vi "Fpga-FPGANic-Top.vi"() -> ()   [LabVIEW 2018]
uses:
  <instrlib>/_niInstr/Network/Ethernet/MAC/CLIP/v1/Resources.ctl
  <vilib>/Platform/TimedLoop/XDataNode/timing_clust.ctl
  <vilib>/Platform/TimedLoop/XDataNode/nitl_modes.ctl
  <vilib>/Platform/TimedLoop/XDataNode/wakeup.ctl
  <instrlib>/_niInstr/Network/Ethernet/MAC/Raw Stream/v1/niInstr Ethernet MAC Raw Stream v1.lvclass
  <instrlib>/_niInstr/Network/Ethernet/Utility/v1/FPGA/Network Data Stream.ctl
  States/FPGANic.Read.States.ctl
  States/FPGANic.Write.States.ctl
  <vilib>/rvi/Emulation/niFpgaSctlEmulationGetInTimedLoop.vi
  <vilib>/rvi/Emulation/niFpgaEmulationReportErrorSimple.vi
  <vilib>/rvi/Emulation/niFpgaGetClockAttributes.vi
  <vilib>/rvi/Emulation/niFpgaCriticalErrorInLSC.vi
  <vilib>/rvi/eio/common/nirviEmuTemplateMethod_errors.vi
  <vilib>/rvi/interface/RandomDataEmulation/niFpgaRandomDataHandleErrors.vi
  <vilib>/rvi/DataTransferAndStorage/Container/Common/niFpgaContainerGetUniqueNameForEmu.vi
  <vilib>/rvi/DataTransferAndStorage/Container/Common/niFpgaContainerSetEmuInfo.vi
  <vilib>/rvi/eio/common/nirviEmuReportErrorAndStop.vi
  <vilib>/rvi/DataTransferAndStorage/Container/Common/niFpgaContainerExecOnDevCompGetState.vi
  <vilib>/rvi/Emulation/niFpgaEmulationIsFPGAContextNoSignature.vi
  <vilib>/rvi/errors/niFpgaSetErrorForExecOnDevCompSimple.vi
  <vilib>/rvi/FIFO/Fifo_Resource/nirvififoEmulationSetSize.vi
  <vilib>/rvi/FIFO/Fifo_Resource/nirviFifoEmulationQueueMgr.vi
  <instcachedir>/0/nirviFifoEmulationQueueMgr_E5CAEC123FF24DC58D834DCA3CDAA9B5.lvgen/nirviFifoEmulationQueueMgr_E5CAEC123FF24DC58D834DCA3CDAA9B5_003.vi
  <vilib>/rvi/FIFO/Fifo_Resource/nirvififoEmulationDetermineInputValidOut.vi
  <vilib>/rvi/FIFO/Fifo_Resource/nirvififoEmulationCreateLock.vi
  <vilib>/rvi/Emulation/niFpgaProcessEmulError.vi
  <vilib>/rvi/FIFO/Fifo_Resource/nirvififoEmulationObtainLock.vi
  <vilib>/rvi/FIFO/Fifo_Resource/nirvififoEmulationReleaseLock.vi
  <vilib>/rvi/occurrence/nirviWaitOnOccurrenceBase.vi
  <vilib>/rvi/errors/nirviReportUnexpectedCaseInternalError.vi
  <vilib>/rvi/errors/nirviReportUnexpectedCaseInternalError (U32).vi
  <vilib>/Utility/error.llb/Clear Errors.vi
  <instrlib>/_niInstr/Network/Ethernet/MAC/Raw Stream/v1/Read End of Bad Frame.vi
  <instrlib>/_niInstr/Network/Ethernet/MAC/Raw Stream/v1/Read End of Good Frame.vi
  <instrlib>/_niInstr/Network/Ethernet/MAC/Raw Stream/v1/Read Data Stream.vi
  <instcachedir>/0/nirviFifoEmulationQueueMgr_E5CAEC123FF24DC58D834DCA3CDAA9B5.lvgen/nirviFifoEmulationQueueMgr_E5CAEC123FF24DC58D834DCA3CDAA9B5_006.vi
  <instrlib>/_niInstr/Network/Ethernet/MAC/Raw Stream/v1/Write Data Stream.vi
  <instrlib>/_niInstr/Network/Ethernet/MAC/Raw Stream/v1/Write End of Bad Frame.vi
  <instrlib>/_niInstr/Network/Ethernet/MAC/Raw Stream/v1/Write End of Good Frame.vi
  <vilib>/Platform/TimedLoop/XDataNode/XDataNode.xnode
  <vilib>/eio/EIONode/EIONode.xnode
  <vilib>/rvi/DataTransferAndStorage/Container/XNode/niFpgaContainer.xnode
  <vilib>/rvi/interface/RandomDataEmulation/nirviRandomDataFpgaReadWriteTemplate.vi
  <vilib>/rvi/LocalResourceManager/LocalResourceManager.xnode
  <vilib>/rvi/FIFO/Fifo_Resource/niFpgaFifoEmulationRefIn.vi
  <instrlib>/_niInstr/Network/Ethernet/MAC/CLIP/v1/niInstr Ethernet MAC - CLIP v1.lvclass
  <vilib>/Platform/TimedLoop/XDataNode/XDNodeRunTimeDep.lvlib
  <instrlib>/_niInstr/Network/Ethernet/Utility/v1/FPGA/niInstr Ethernet Utilities FPGA v1.lvlib
panel:
  in  "d_microblaze_i\\reset_rtl":bool=TRUE
  out "GPIO #1 out":u32
  in  "GPIO #1 in":u32
  in  "d_microblaze_i\\AXI_STR_RXD_3_tkeep":u8=15
  out "mgtrefclks_locked":bool
  out "mgtrefclks_valid":bool
  out "posc_complete":bool
  out "sPort0_Power_Good":bool
  out "sPort1_Power_Good":bool
  out "signal_detect_Port0":bool
  out "signal_detect_Port1":bool
  out "aBlockLockPort0":bool
  out "aBlockLockPort1":bool
  out "GPIO #2 out":u32
  in  "GPIO #2 in":u32
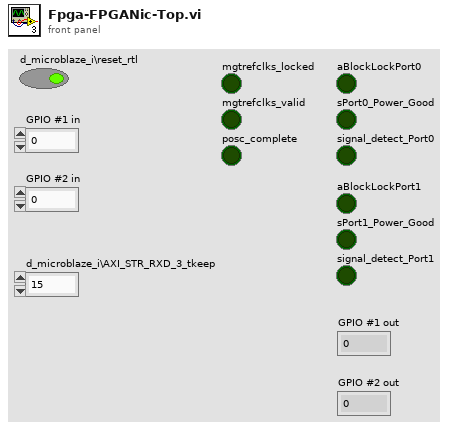
[diagram p1: front panel]
types:
  T1 = typedef "niInstr Ethernet MAC - CLIP v1.lvclass/Resources.ctl" = cluster{"RX":cluster{"TData":refnum<k21>, "TValid":refnum<k21>, "TKeep":refnum<k21>, "TLast":refnum<k21>, "TUser":refnum<k21>}, "TX":cluster{"TData":refnum<k21>, "TValid":refnum<k21>, "TKeep":refnum<k21>, "TLast":refnum<k21>, "TReady":refnum<k21>}, "Pause resources":cluster{"cPauseValuePort":refnum<k21>, "cPauseReqPort":refnum<k21>}, "MAC Clock":refnum<k21>}
  T2 = typedef "XDNodeRunTimeDep.lvlib/timing_clust.ctl" = cluster{"Expected End [f-1]":u64, "Actual End [f-1]":u64, "Finished Late? [f-1]":bool, "Expected End [i-1]":u64, "Actual End [i-1]":u64, "Finished Late? [i-1]":bool, "Expected Start [i]":u64, "Actual Start [i]":u64, "Expected Start [f]":u64, "Actual Start [f]":u64, "Source Name":string, "Structure Name":string, "Period":i64, "Deadline":i64, "Offset":i64, "Start":i64, "Priority":i32, "Timeout":i32, "Mode":T3, "Wakeup Reason":T4, "Error":errorcluster, "Source Type":string, "Secondary Source Type":string, "Global End Time":u64, "Global Start Time":u64, "Frame Duration":u64, "Iteration Duration":u64, "Assigned CPU":i32, "I/O Scan Engine Mode":u32}
  T3 = typedef "XDNodeRunTimeDep.lvlib/nitl_modes.ctl" = enum32{"No Change", "Process missed periods, maintain original phase", "Discard missed periods, maintain original phase", "Process missed periods, ignore original phase", "Discard missed periods, ignore original phase"}
  T4 = typedef "XDNodeRunTimeDep.lvlib/wakeup.ctl" = enum32{"Normal", "Aborted", "Asynchronous wakeup", "Timing source error", "Timed loop error", "Timeout"}
  T5 = typedef "niInstr Ethernet Utilities FPGA v1.lvlib/Network Data Stream.ctl" = cluster{"data":u8[], "data valid":bool, "byte enables":bool[]}
  T6 = cluster{"tdata[63:0]":u64, "tlast":bool, "tkeep[7:0]":bool[], "EndOfGoodFrame":bool, "EndOfBadFrame":bool}
  T7 = typedef "FPGANic.Write.States.ctl" = enum16{"Read-Top", "Read-Bottom"}
  T8 = typedef "FPGANic.Read.States.ctl" = enum16{"Read-Top", "Read-Bottom", "Append-Size"}
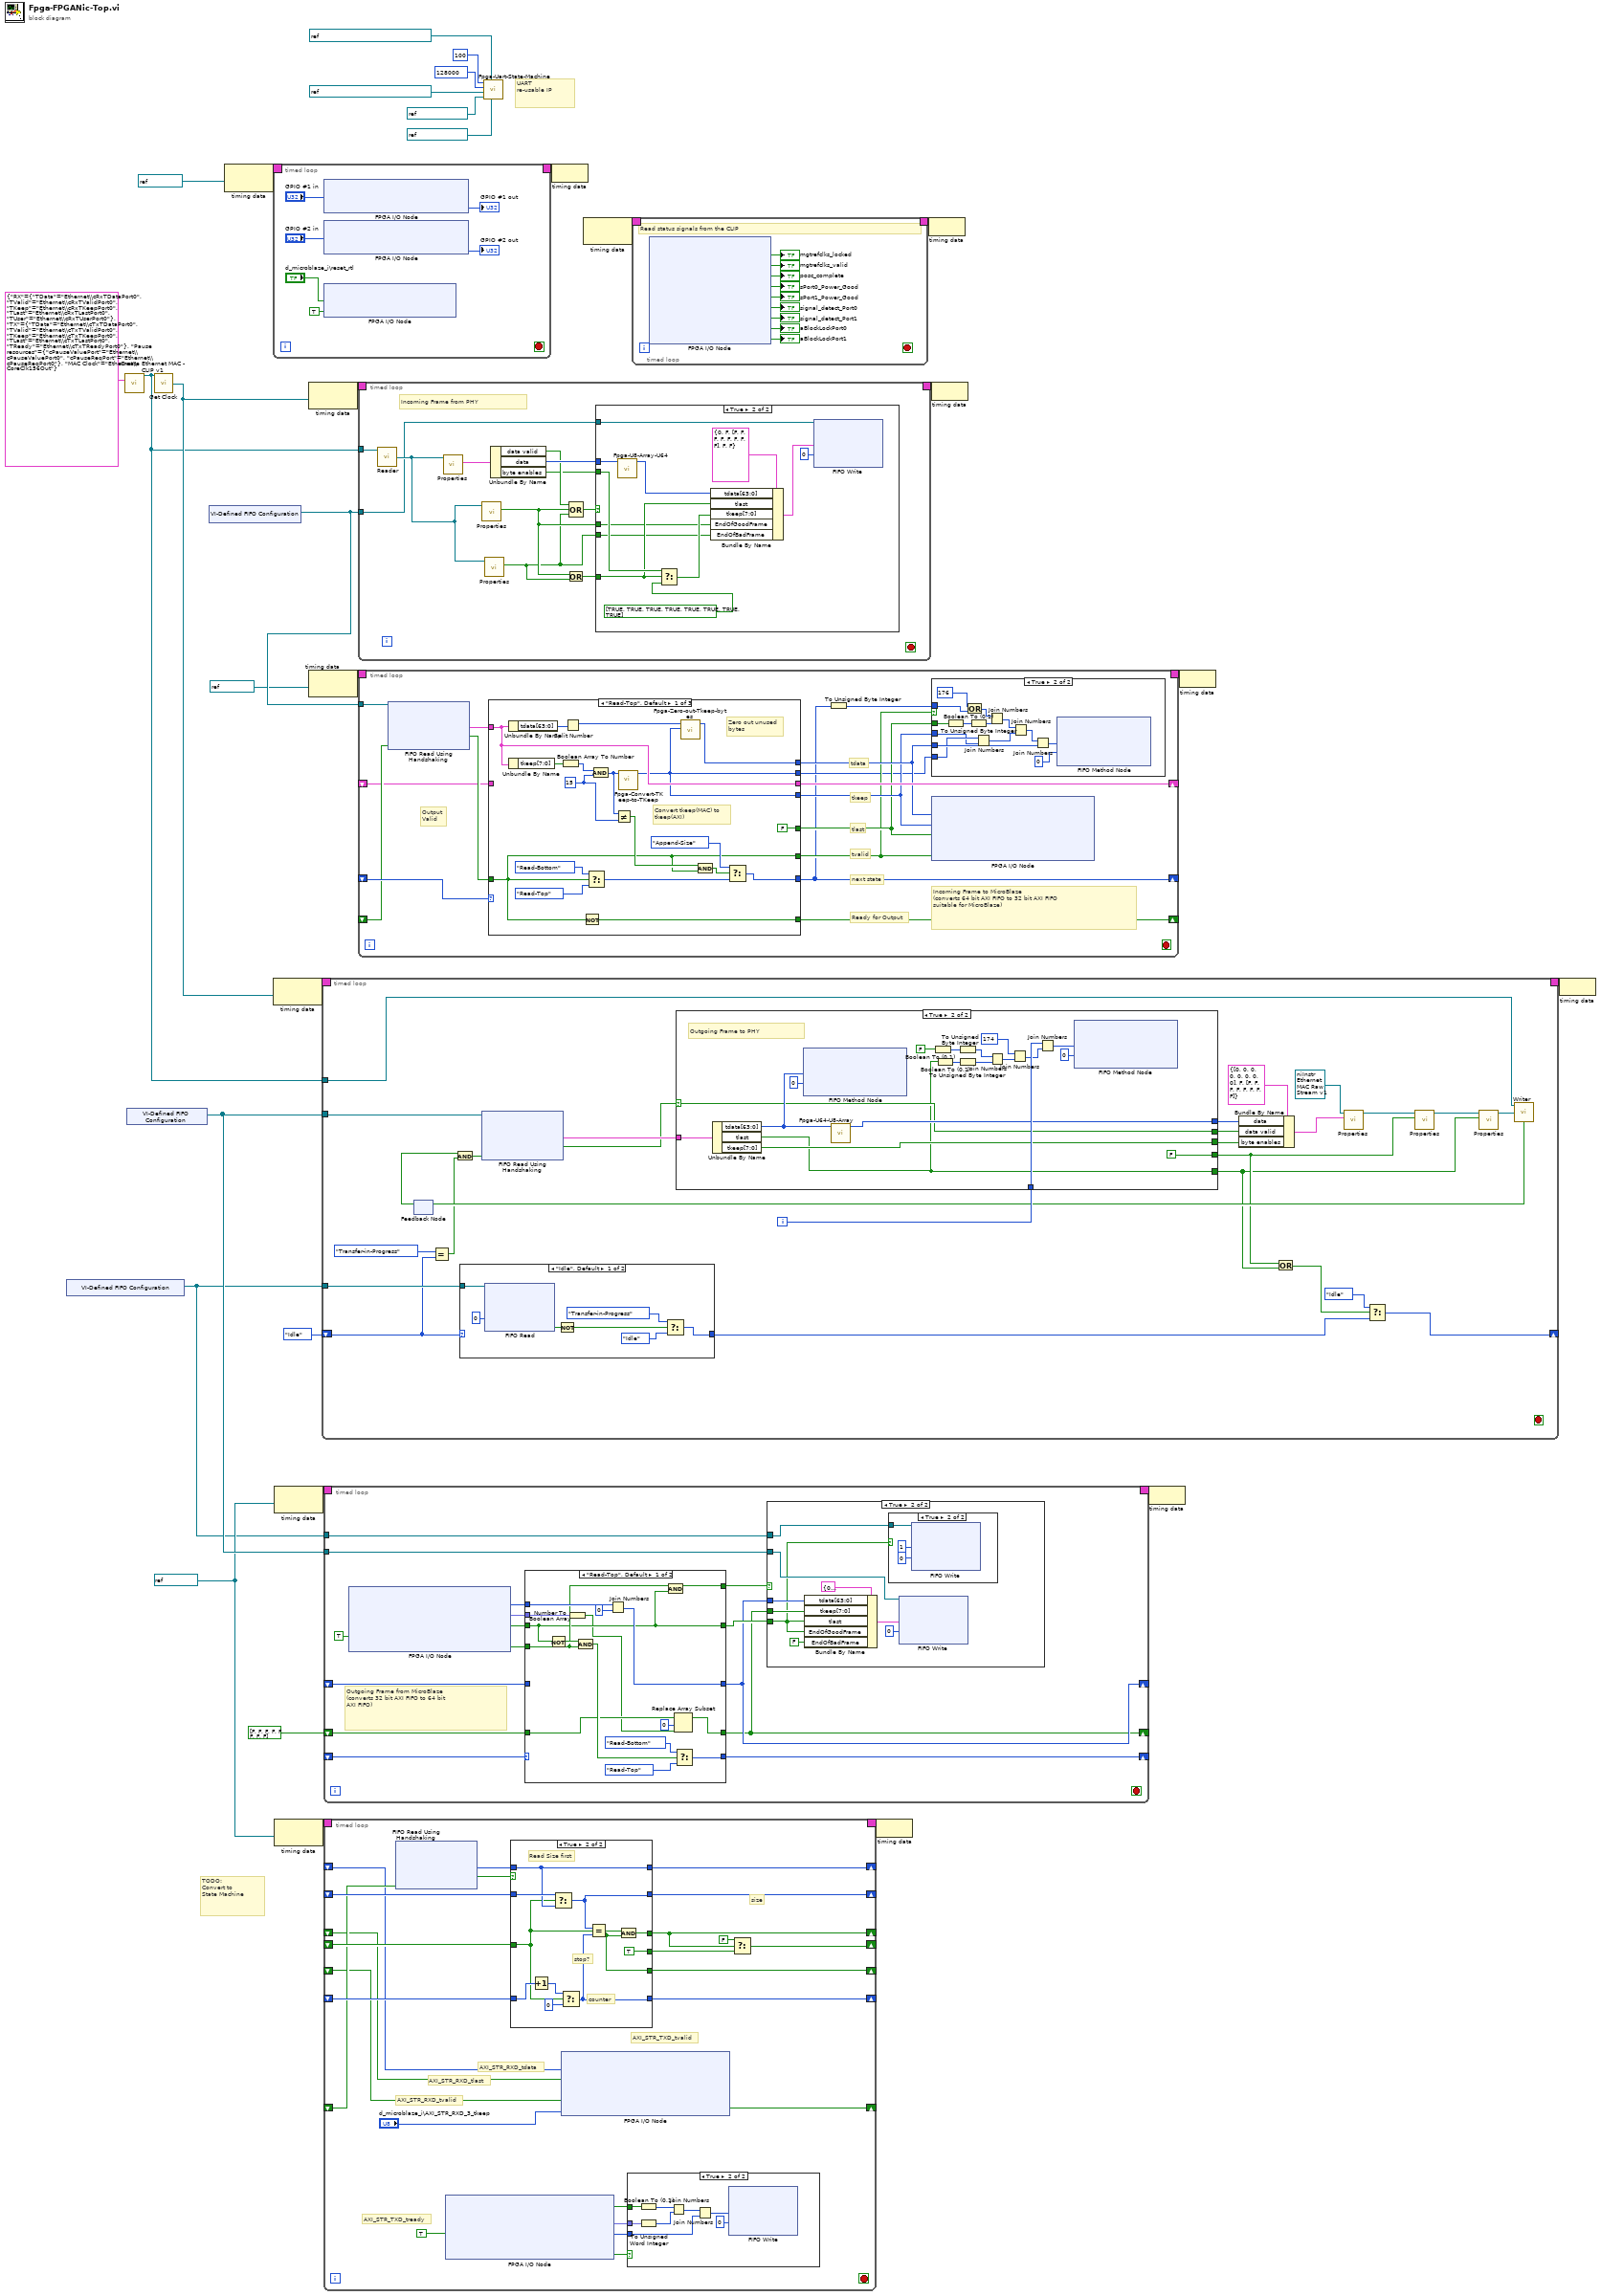
[diagram p0: block diagram]
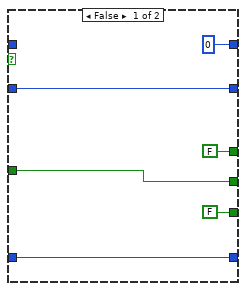
[diagram p3: hidden frame]
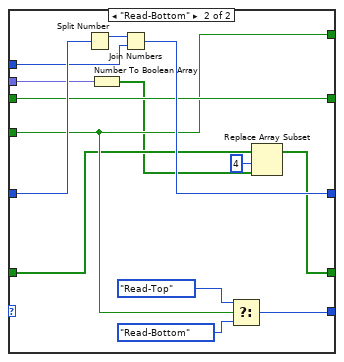
[diagram p4: hidden frame]
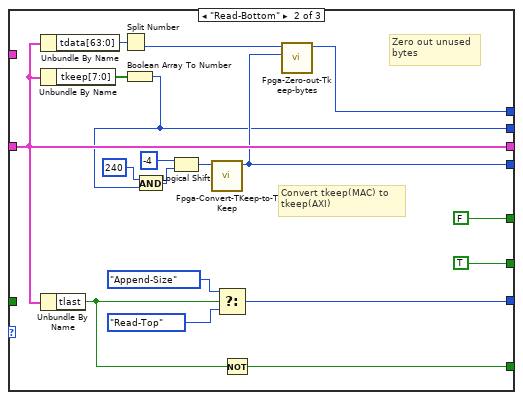
[diagram p7: hidden frame]
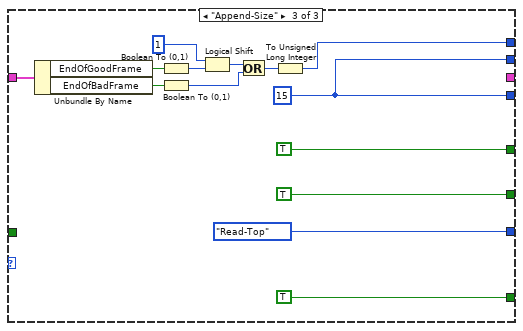
[diagram p8: hidden frame]
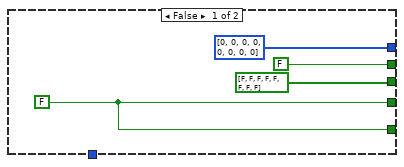
[diagram p11: hidden frame]
diagram:
  w8 = u32 128000 items=["110"=110, "300"=300, "1200"=1200, "2400"=2400, "4800"=4800, "9600"=9600, "19200"=19200, "38400"=38400, "57600"=57600, "115200"=115200, "128000"=128000, "230400"=230400, "460800"=460800, "921600"=921600] ("Baud Rate")
  w10 = refnum<k21> "100MHz" ("Source Name")
  # "UART\nre-usable IP"
  # "TODO:\nConvert to \nState Machine"
  n1 = xnode "VI-Defined FIFO Configuration"() -> ("FIFO Out"=w2:refnum<k21>)
  n2 = call <instrlib>:"Create Ethernet MAC - CLIP v1.vi"("Ethernet AXI4-S Resources"=T1 {"RX"={"TData"="Ethernet\\cRxTDataPort0", "TValid"="Ethernet\\cRxTValidPort0", "TKeep"="Ethernet\\cRxTKeepPort0", "TLast"="Ethernet\\cRxTLastPort0", "TUser"="Ethernet\\cRxTUserPort0"}, "TX"={"TData"="Ethernet\\cTxTDataPort0", "TValid"="Ethernet\\cTxTValidPort0", "TKeep"="Ethernet\\cTxTKeepPort0", "TLast"="Ethernet\\cTxTLastPort0", "TReady"="Ethernet\\cTxTReadyPort0"}, "Pause resources"={"cPauseValuePort"="Ethernet\\cPauseValuePort0", "cPauseReqPort"="Ethernet\\cPauseReqPort0"}, "MAC Clock"="Ethernet\\CoreClk156Out"}) -> ("niInstr Ethernet MAC - CLIP v1.lvclass out"=w20:refnum<class "niInstr Ethernet MAC - CLIP v1.lvclass">)  [unwired: 14 in]
  n3 = xnode "VI-Defined FIFO Configuration"() -> ("FIFO Out"=w13:refnum<k21>)
  n4 = call-dynamic "Get Clock.vi"("niInstr Ethernet MAC - CLIP v1.lvclass"=w20) -> ("MAC Clock"=w21:refnum<k21>)  [unwired: 14 in]
  n5 = xnode "VI-Defined FIFO Configuration"() -> ("FIFO Out"=w17:refnum<k21>)
  n6 = node-c288(refnum<k21> "100MHz" ("Source Name")) -> (w31:T2)
  n7 = node-c288(w21) -> (w24:T2)
  n8 = timed-loop {
    timing: w31 -> [_]
    timing-out: [_] -> w30
    stop <- _ stop-if-true
    n9 = xnode "FPGA I/O Node"("UserRTL_microblaze\\gpio_rtl_tri_i"="GPIO #1 in") -> ("UserRTL_microblaze\\gpio_rtl_0_tri_o"=→"GPIO #1 out":u32)  [unwired: 2 in, 2 out]
    n10 = xnode "FPGA I/O Node"("UserRTL_microblaze\\gpio_rtl_1_tri_i"="GPIO #2 in") -> ("UserRTL_microblaze\\gpio_rtl_2_tri_o"=→"GPIO #2 out":u32)  [unwired: 2 in, 2 out]
    n11 = xnode "FPGA I/O Node"("UserRTL_microblaze\\reset_rtl"="d_microblaze_i\\reset_rtl", "UserRTL_microblaze\\uart_rtl_rxd"=TRUE ("d_microblaze_i\\uart_rtl_rxd")) -> ()  [unwired: 2 in, 2 out]
  }
  n12 = node-c288(w10) -> (w15:T2)
  n13 = node-c288(w10) -> (w12:T2)
  n14 = node-c288(w21) -> (w28:T2)
  n15 = node-c288(refnum<k21> "100MHz" ("Source Name")) -> (w19:T2)
  n16 = timed-loop {
    timing: w24 -> [_]
    timing-out: [_] -> w23
    tunnel: w20 -> [w61]
    tunnel: w13 -> [w66]
    tunnel: w2 -> [w51]
    shift-right: [w40] -> _
    shift-left: enum16{"Idle", "Transfer-in-Progress"}."Idle" ("Enum") -> [w50]
    i -> [w63]
    stop <- _ stop-if-true
    n17 = feedback #1() -> (w47:bool)  [unwired: 1 in]
    n18 = Equal?(x=enum16{"Idle", "Transfer-in-Progress"}."Transfer-in-Progress", y=w50) -> (x = y?=w48:bool)
    n19 = And(x=w47, y=w48) -> (x .and. y?=w46:bool)
    n20 = case shown="\"Idle\", Default" w50 {
      selector: w50 -> [_ w74]
      tunnel: w51 -> [w73 _]
      tunnel: [w69 w74] -> w42
      frame "Idle", Default {
        n21 = xnode ("FIFO Read")("Timeout"=0, "FIFO In"=w73) -> ("Timed Out?"=w67:bool)  [unwired: 2 out]
        n22 = Not(x=w67) -> (.not. x?=w70:bool)
        n23 = Select(t=enum16{"Idle", "Transfer-in-Progress"}."Transfer-in-Progress" ("Enum"), s=w70, f=enum16{"Idle", "Transfer-in-Progress"}."Idle" ("Enum")) -> (s? t:f=w69:enum16{"Idle", "Transfer-in-Progress"})
      }
      frame "Transfer-in-Progress" {
      }
    }
    n24 = xnode ("FIFO Read Using Handshaking")("Ready for Output"=w46, "FIFO In"=w66) -> ("Element"=w65:T6, "Output Valid"=w64:bool)  [unwired: 1 out]
    n25 = case shown="True" w64 {
      selector: w64 -> [_ w82]
      tunnel: w65 -> [_ w97]
      tunnel: w63 -> [_ w96]
      tunnel: [w78 FALSE ("End of Good Frame")] -> w45
      tunnel: [w78 w79] -> w44
      tunnel: [u8[] [0, 0, 0, 0, 0, 0, 0, 0] ("U8[] out") w83] -> w57
      tunnel: [FALSE w82] -> w56
      tunnel: [bool[] [FALSE, FALSE, FALSE, FALSE, FALSE, FALSE, FALSE, FALSE] ("tkeep[7:0]") w81] -> w55
      frame False {
        w78 = FALSE ("End of Good Frame")
      }
      frame True {
        # "Outgoing Frame to PHY"
        n26 = Unbundle By Name(w97) -> ("tdata[63:0]"=w85:u64, "tlast"=w79:bool, "tkeep[7:0]"=w81:bool[])
        n27 = xnode ("FIFO Method Node")("Element"=w85, "Timeout"=0) -> ()  [unwired: 1 in, 2 out]
        n28 = call "Fpga-U64-U8-Array.vi"("U64 in"=w85) -> ("U8[] out"=w83:u8[])  [unwired: 10 in]
        n29 = Boolean To (0,1)(Boolean=FALSE) -> (0, 1=w87:i16)
        n30 = Boolean To (0,1)(Boolean=w79) -> (0, 1=w84:i16)
        n31 = To Unsigned Byte Integer(number=w87) -> (unsigned 8bit integer=w88:u8)
        n32 = To Unsigned Byte Integer(number=w84) -> (unsigned 8bit integer=w89:u8)
        n33 = Join Numbers(hi=w88, lo=w89) -> ((hi.lo)=w90:u16)
        n34 = Join Numbers(hi=u16 174, lo=w90) -> ((hi.lo)=w91:u32)
        n35 = Join Numbers(hi=w96, lo=w91) -> ((hi.lo)=w92:u64)
        n36 = xnode ("FIFO Method Node")("Element"=w92, "Timeout"=0) -> ()  [unwired: 1 in, 2 out]
      }
    }
    n37 = Bundle By Name(cluster=T5 {"data"=[0, 0, 0, 0, 0, 0, 0, 0], "data valid"=FALSE, "byte enables"=[FALSE, FALSE, FALSE, FALSE, FALSE, FALSE, FALSE, FALSE]} ("Data Stream"), "data"=w57, "data valid"=w56, "byte enables"=w55) -> (w53:T5)
    n38 = Or(x=w45, y=w44) -> (x .or. y?=w43:bool)
    n39 = call-poly <instrlib>:"Properties.vi"("Data Stream"=w53, "niInstr Ethernet MAC Data Stream v1 in"=refnum<class "niInstr Ethernet MAC Raw Stream v1.lvclass"> refnum) -> ("niInstr Ethernet MAC Data Stream v1 out"=w58:refnum<class "niInstr Ethernet MAC Raw Stream v1.lvclass">)  [unwired: 9 in]
    n40 = Select(t=enum16{"Idle", "Transfer-in-Progress"}."Idle" ("Enum"), s=w43, f=w42) -> (s? t:f=w40:enum16{"Idle", "Transfer-in-Progress"})
    n41 = call-poly <instrlib>:"Properties.vi"("End of Bad Frame"=w45, "niInstr Ethernet MAC Data Stream v1 in"=w58) -> ("niInstr Ethernet MAC Data Stream v1 out"=w60:refnum<class "niInstr Ethernet MAC Raw Stream v1.lvclass">)  [unwired: 9 in]
    n42 = call-poly <instrlib>:"Properties.vi"("End of Good Frame"=w44, "niInstr Ethernet MAC Data Stream v1 in"=w60) -> ("niInstr Ethernet MAC Data Stream v1 out"=w59:refnum<class "niInstr Ethernet MAC Raw Stream v1.lvclass">)  [unwired: 9 in]
    n43 = call-dynamic "Writer.vi"("niInstr Ethernet MAC v1.lvclass"=w61, "niInstr Ethernet MAC Raw Stream v1.lvclass"=w59) -> ("ready for input?"=w62:bool)  [unwired: 12 in, 1 out]
    n44 = feedback-in #1(w62) -> ()
  }
  n45 = timed-loop {
    timing: w15 -> [_]
    timing-out: [_] -> w14
    tunnel: w13 -> [w113]
    shift-right: [w111] -> _
    shift-left: _ -> [w112]
    shift-right: [w103] -> _
    shift-left: _ -> [w107]
    shift-right: [w101] -> _
    shift-left: bool[] [FALSE, FALSE, FALSE, FALSE, FALSE, FALSE, FALSE, FALSE] ("Boolean array") -> [w102]
    tunnel: w2 -> [w100]
    stop <- _ stop-if-true
    # "Outgoing Frame from MicroBlaze\n(converts 32 bit AXI FIFO to 64 bit\nAXI FIFO)"
    n46 = xnode "FPGA I/O Node"("UserRTL_microblaze\\AXI_STR_TXD_tready"=TRUE ("d_microblaze_i\\AXI_STR_TXD_2_tready")) -> ("UserRTL_microblaze\\AXI_STR_TXD_tdata"=w110:u32, "UserRTL_microblaze\\AXI_STR_TXD_tkeep"=w104:fxp<+,4,4>, "UserRTL_microblaze\\AXI_STR_TXD_tlast"=w108:bool, "UserRTL_microblaze\\AXI_STR_TXD_tvalid"=w109:bool)  [unwired: 5 in, 5 out]
    n47 = case shown="\"Read-Top\", Default" w112 {
      tunnel: [w128 w142] -> w111
      tunnel: w110 -> [w127 w138]
      tunnel: w109 -> [w122 w136]
      tunnel: [w125 w141] -> w103
      tunnel: w108 -> [w120 w137]
      tunnel: [w120 w137] -> w106
      tunnel: w107 -> [_ w140]
      tunnel: [w121 w136] -> w105
      tunnel: w104 -> [w119 w135]
      tunnel: w102 -> [w117 w133]
      tunnel: [w115 w134] -> w101
      frame "Read-Top", Default {
        n48 = Not(x=w120) -> (.not. x?=w124:bool)
        n49 = Number To Boolean Array(number=w119) -> (Boolean array=w116:bool[])
        n50 = And(x=w124, y=w122) -> (x .and. y?=w123:bool)
        n51 = Join Numbers(hi=w127, lo=u32 0) -> ((hi.lo)=w125:u64)
        n52 = And(x=w122, y=w120) -> (x .and. y?=w121:bool)
        n53 = Replace Array Subset(array=w117, new element=w116, index=0) -> (w115:bool[])
        n54 = Select(t=FPGANic.Write.States."Read-Bottom" ("Enum"), s=w123, f=FPGANic.Write.States."Read-Top" ("Enum")) -> (s? t:f=w128:T7)
      }
      frame "Read-Bottom" {
        n55 = Split Number(x=w140) -> (hi(x)=w139:u32)  [unwired: 1 out]
        n56 = Number To Boolean Array(number=w135) -> (Boolean array=w132:bool[])
        n57 = Join Numbers(hi=w139, lo=w138) -> ((hi.lo)=w141:u64)
        n58 = Select(t=FPGANic.Write.States."Read-Top" ("Enum"), s=w136, f=FPGANic.Write.States."Read-Bottom" ("Enum")) -> (s? t:f=w142:T7)
        n59 = Replace Array Subset(array=w133, new element=w132, index=4) -> (w134:bool[])
      }
    }
    n60 = case shown="True" w105 {
      tunnel: w113 -> [_ w146]
      tunnel: w103 -> [_ w150]
      tunnel: w106 -> [_ w145]
      tunnel: w101 -> [_ w148]
      tunnel: w100 -> [_ w147]
      frame False {
      }
      frame True {
        n61 = Bundle By Name(cluster=T6 {"tdata[63:0]"=0, "tlast"=FALSE, "tkeep[7:0]"=[FALSE, FALSE, FALSE, FALSE, FALSE, FALSE, FALSE, FALSE], "EndOfGoodFrame"=FALSE, "EndOfBadFrame"=FALSE} ("AXI4-Pins"), "tdata[63:0]"=w150, "tkeep[7:0]"=w148, "tlast"=w145, "EndOfGoodFrame"=w145, "EndOfBadFrame"=FALSE) -> (w152:T6)
        n62 = case shown="True" w145 {
          tunnel: w147 -> [_ w156]
          frame False {
          }
          frame True {
            n63 = xnode ("FIFO Write")("Element"=u16 1, "Timeout"=0, "FIFO In"=w156) -> ()  [unwired: 2 out]
          }
        }
        n64 = xnode ("FIFO Write")("Element"=w152, "Timeout"=0, "FIFO In"=w146) -> ()  [unwired: 2 out]
      }
    }
  }
  n65 = timed-loop {
    timing: w12 -> [_]
    timing-out: [_] -> w11
    shift-right: [w166] -> _
    shift-left: _ -> [w181]
    shift-right: [w178] -> _
    shift-left: _ -> [w180]
    shift-right: [w176] -> _
    shift-left: _ -> [w177]
    shift-right: [w164] -> _
    shift-left: _ -> [w171]
    shift-right: [w163] -> _
    shift-left: _ -> [w175]
    shift-right: [w174] -> _
    shift-left: _ -> [w173]
    shift-right: [w165] -> _
    shift-left: _ -> [w172]
    stop <- _ stop-if-true
    # "size"
    # "AXI_STR_TXD_tvalid"
    # "AXI_STR_TXD_tready"
    # "AXI_STR_RXD_tvalid"
    # "AXI_STR_RXD_tlast"
    # "AXI_STR_RXD_tdata"
    n66 = xnode ("FIFO Read Using Handshaking")("Ready for Output"=w175) -> ("Element"=w179:u64, "Output Valid"=w182:bool)  [unwired: 1 in, 1 out]
    n67 = xnode "FPGA I/O Node"("UserRTL_microblaze\\AXI_STR_TXD_1_tready"=TRUE ("d_microblaze\\AXI_STR_TXD_tready")) -> ("UserRTL_microblaze\\AXI_STR_TXD_1_tlast"=w160:bool, "UserRTL_microblaze\\AXI_STR_TXD_1_tkeep"=w159:fxp<+,4,4>, "UserRTL_microblaze\\AXI_STR_TXD_1_tdata"=w161:u32, "UserRTL_microblaze\\AXI_STR_TXD_1_tvalid"=w169:bool)  [unwired: 5 in, 5 out]
    n68 = case shown="True" w182 {
      tunnel: w181 -> [w195 w197]
      tunnel: [w195 TRUE ("Size\nRead?")] -> w167
      tunnel: w180 -> [w196 w207]
      tunnel: w179 -> [_ w202]
      tunnel: [w196 w201] -> w178
      tunnel: w177 -> [w194 w206]
      tunnel: [w194 w200] -> w176
      tunnel: [FALSE ("Size\nRead?") w197] -> w164
      tunnel: [u64 0 ("Element") w202] -> w174
      tunnel: [FALSE w198] -> w165
      frame False {
      }
      frame True {
        # "Read Size first"
        # "stop?"
        # "counter"
        n69 = Increment(x=w206) -> (x+1=w204:u64)
        n70 = Select(t=w207, s=w197, f=w202) -> (s? t:f=w201:u64)
        n71 = Select(t=w204, s=w197, f=u64 0) -> (s? t:f=w200:u64)
        n72 = Equal?(x=w201, y=w200) -> (x = y?=w199:bool)
        n73 = And(x=w199, y=w197) -> (x .and. y?=w198:bool)
      }
    }
    n74 = xnode "FPGA I/O Node"("UserRTL_microblaze\\AXI_STR_RXD_1_tdata"=w173, "UserRTL_microblaze\\AXI_STR_RXD_1_tlast"=w172, "UserRTL_microblaze\\AXI_STR_RXD_1_tvalid"=w171, "UserRTL_microblaze\\AXI_STR_RXD_1_tkeep"="d_microblaze_i\\AXI_STR_RXD_3_tkeep") -> ("UserRTL_microblaze\\AXI_STR_RXD_1_tready"=w163:bool)  [unwired: 5 in, 5 out]
    n75 = case shown="True" w169 {
      tunnel: w161 -> [_ w189]
      tunnel: w160 -> [_ w185]
      tunnel: w159 -> [_ w184]
      frame False {
      }
      frame True {
        n76 = Boolean To (0,1)(Boolean=w185) -> (0, 1=w186:i16)
        n77 = To Unsigned Word Integer(number=w184) -> (unsigned 16bit integer=w183:u16)
        n78 = Join Numbers(hi=w186, lo=w183) -> ((hi.lo)=w187:u32)
        n79 = Join Numbers(hi=w187, lo=w189) -> ((hi.lo)=w188:u64)
        n80 = xnode ("FIFO Write")("Element"=w188, "Timeout"=0) -> ()  [unwired: 1 in, 2 out]
      }
    }
    n81 = Select(t=FALSE, s=w165, f=w167) -> (s? t:f=w166:bool)
  }
  n82 = timed-loop {
    timing: w28 -> [_]
    timing-out: [_] -> w27
    tunnel: w20 -> [w220]
    tunnel: w17 -> [w216]
    stop <- _ stop-if-true
    # "Incoming Frame from PHY"
    n83 = call-dynamic "Reader.vi"("niInstr Ethernet MAC - CLIP v1.lvclass 2"=w220) -> ("niInstr Ethernet MAC Raw Stream v1.lvclass"=w217:refnum<class "niInstr Ethernet MAC Raw Stream v1.lvclass">)  [unwired: 13 in, 1 out]
    n84 = call-poly <instrlib>:"Properties.vi"("niInstr Ethernet MAC Data Stream v1 in"=w217) -> ("Data Stream"=w219:T5)  [unwired: 9 in, 1 out]
    n85 = call-poly <instrlib>:"Properties.vi"("niInstr Ethernet MAC Data Stream v1 in"=w217) -> ("End of Good Frame"=w211:bool)  [unwired: 9 in, 1 out]
    n86 = call-poly <instrlib>:"Properties.vi"("niInstr Ethernet MAC Data Stream v1 in"=w217) -> ("End of Bad Frame"=w210:bool)  [unwired: 9 in, 1 out]
    n87 = Unbundle By Name(w219) -> ("data valid"=w215:bool, "data"=w218:u8[], "byte enables"=w212:bool[])
    n88 = Or(x=w211, y=w210) -> (x .or. y?=w213:bool)
    n89 = Compound Arithmetic op=OR(w215, w211, w210) -> (w214:bool)
    n90 = case shown="True" w214 {
      tunnel: w218 -> [_ w230]
      tunnel: w216 -> [_ w231]
      tunnel: w213 -> [_ w224]
      tunnel: w212 -> [_ w225]
      tunnel: w211 -> [_ w223]
      tunnel: w210 -> [_ w222]
      frame False {
      }
      frame True {
        n91 = call "Fpga-U8-Array-U64.vi"("U8[] in"=w230) -> ("U64 out"=w227:u64)  [unwired: 10 in]
        n92 = Select(t=w225, s=w224, f=bool[] [TRUE, TRUE, TRUE, TRUE, TRUE, TRUE, TRUE, TRUE] ("s? t:f")) -> (s? t:f=w226:bool[])
        n93 = Bundle By Name(cluster=T6 {"tdata[63:0]"=0, "tlast"=FALSE, "tkeep[7:0]"=[FALSE, FALSE, FALSE, FALSE, FALSE, FALSE, FALSE, FALSE], "EndOfGoodFrame"=FALSE, "EndOfBadFrame"=FALSE} ("Element"), "tdata[63:0]"=w227, "tlast"=w224, "tkeep[7:0]"=w226, "EndOfGoodFrame"=w223, "EndOfBadFrame"=w222) -> (w228:T6)
        n94 = xnode ("FIFO Write")("Element"=w228, "Timeout"=0, "FIFO In"=w231) -> ()  [unwired: 2 out]
      }
    }
  }
  n95 = timed-loop {
    timing: w19 -> [_]
    timing-out: [_] -> w18
    tunnel: w17 -> [w249]
    shift-right: [w246] -> _
    shift-left: _ -> [w242]
    shift-right: [w236] -> _
    shift-left: _ -> [w245]
    shift-right: [w244] -> _
    shift-left: _ -> [w243]
    stop <- _ stop-if-true
    # "tdata"
    # "Incoming Frame to MicroBlaze\n(converts 64 bit AXI FIFO to 32 bit AXI FIFO\nsuitable for MicroBlaze)"
    # "Output\nValid"
    # "Ready for Output"
    # "next state"
    # "tkeep"
    # "tlast"
    # "tvalid"
    n96 = xnode ("FIFO Read Using Handshaking")("Ready for Output"=w243, "FIFO In"=w249) -> ("Element"=w247:T6, "Output Valid"=w248:bool)  [unwired: 1 out]
    n97 = case shown="\"Read-Top\", Default" w245 {
      tunnel: w248 -> [w250 _ _]
      tunnel: w247 -> [w264 _ _]
      tunnel: [w255 w276 w291] -> w241
      tunnel: [w257 w283 FPGANic.Read.States."Read-Top" ("Enum")] -> w236
      tunnel: [w250 TRUE ("Output Valid") TRUE ("Output Valid")] -> w238
      tunnel: [FALSE FALSE TRUE] -> w239
      tunnel: [w253 w275 w287] -> w240
      tunnel: [w264 w284 _] -> w246
      tunnel: [w265 w278 TRUE ("tlast")] -> w244
      tunnel: w242 -> [_ w284 w294]
      tunnel: [w253 w271 w287] -> w237
      frame "Read-Top", Default {
        w260 = u8 15 ("x")
        # "Convert tkeep(MAC) to\ntkeep(AXI)"
        # "Zero out unused\nbytes"
        n98 = Unbundle By Name(w264) -> ("tdata[63:0]"=w268:u64)
        n99 = Unbundle By Name(w264) -> ("tkeep[7:0]"=w263:bool[])
        n100 = Boolean Array To Number(Boolean array=w263) -> (number=w262:u8)
        n101 = Split Number(x=w268) -> (hi(x)=w254:u32)  [unwired: 1 out]
        n102 = Not(x=w250) -> (.not. x?=w265:bool)
        n103 = Select(t=FPGANic.Read.States."Read-Bottom" ("Enum"), s=w250, f=FPGANic.Read.States."Read-Top" ("Enum")) -> (s? t:f=w259:T8)
        n104 = And(x=w262, y=w260) -> (x .and. y?=w261:u8)
        n105 = Not Equal?(x=w261, y=w260) -> (x != y?=w251:bool)
        n106 = call "Fpga-Convert-TKeep-to-TKeep.vi"("tkeep (MAC)"=w261) -> ("tkeep (MicroBlaze)"=w253:u8)  [unwired: 10 in]
        n107 = call "Fpga-Zero-out-Tkeep-bytes.vi"("tkeep (MAC)"=w253, "data_in"=w254) -> ("data_out"=w255:u32)  [unwired: 9 in]
        n108 = And(x=w251, y=w250) -> (x .and. y?=w252:bool)
        n109 = Select(t=FPGANic.Read.States."Append-Size" ("Enum"), s=w252, f=w259) -> (s? t:f=w257:T8)
      }
      frame "Read-Bottom" {
        # "Convert tkeep(MAC) to\ntkeep(AXI)"
        # "Zero out unused\nbytes"
        n110 = Unbundle By Name(w284) -> ("tdata[63:0]"=w286:u64)
        n111 = Unbundle By Name(w284) -> ("tkeep[7:0]"=w285:bool[])
        n112 = Unbundle By Name(w284) -> ("tlast"=w280:bool)
        n113 = Split Number(x=w286) -> (lo(x)=w277:u32)  [unwired: 1 out]
        n114 = Boolean Array To Number(Boolean array=w285) -> (number=w271:u8)
        n115 = And(x=u8 240, y=w271) -> (x .and. y?=w272:u8)
        n116 = Logical Shift(y=i16 -4, x=w272) -> (x << y=w270:u8)
        n117 = call "Fpga-Convert-TKeep-to-TKeep.vi"("tkeep (MAC)"=w270) -> ("tkeep (MicroBlaze)"=w275:u8)  [unwired: 10 in]
        n118 = Select(t=FPGANic.Read.States."Append-Size" ("Enum"), s=w280, f=FPGANic.Read.States."Read-Top" ("Enum")) -> (s? t:f=w283:T8)
        n119 = Not(x=w280) -> (.not. x?=w278:bool)
        n120 = call "Fpga-Zero-out-Tkeep-bytes.vi"("tkeep (MAC)"=w275, "data_in"=w277) -> ("data_out"=w276:u32)  [unwired: 9 in]
      }
      frame "Append-Size" {
        w287 = u8 15 ("t")
        n121 = Unbundle By Name(w294) -> ("EndOfGoodFrame"=w293:bool, "EndOfBadFrame"=w292:bool)
        n122 = Boolean To (0,1)(Boolean=w293) -> (0, 1=w298:i16)
        n123 = Boolean To (0,1)(Boolean=w292) -> (0, 1=w295:i16)
        n124 = Logical Shift(y=i16 1, x=w298) -> (x << y=w296:i16)
        n125 = Or(x=w296, y=w295) -> (x .or. y?=w299:i16)
        n126 = To Unsigned Long Integer(number=w299) -> (unsigned 32bit integer=w291:u32)
      }
    }
    n127 = To Unsigned Byte Integer(number=w236) -> (unsigned 8bit integer=w235:u8)
    n128 = case shown="True" w238 {
      tunnel: w241 -> [_ w312]
      tunnel: w240 -> [_ w304]
      tunnel: w239 -> [_ w310]
      tunnel: w237 -> [_ w305]
      tunnel: w235 -> [_ w301]
      frame False {
      }
      frame True {
        n129 = Boolean To (0,1)(Boolean=w310) -> (0, 1=w309:i16)
        n130 = Or(x=u8 176 ("hi"), y=w301) -> (x .or. y?=w302:u8)
        n131 = To Unsigned Byte Integer(number=w309) -> (unsigned 8bit integer=w308:u8)
        n132 = Join Numbers(hi=w305, lo=w304) -> ((hi.lo)=w306:u16)
        n133 = Join Numbers(hi=w302, lo=w308) -> ((hi.lo)=w307:u16)
        n134 = Join Numbers(hi=w307, lo=w306) -> ((hi.lo)=w311:u32)
        n135 = Join Numbers(hi=w311, lo=w312) -> ((hi.lo)=w313:u64)
        n136 = xnode ("FIFO Method Node")("Element"=w313, "Timeout"=0) -> ()  [unwired: 1 in, 2 out]
      }
    }
    n137 = xnode "FPGA I/O Node"("UserRTL_microblaze\\AXI_STR_RXD_tdata"=w241, "UserRTL_microblaze\\AXI_STR_RXD_tkeep"=w240, "UserRTL_microblaze\\AXI_STR_RXD_tlast"=w239, "UserRTL_microblaze\\AXI_STR_RXD_tvalid"=w238) -> ()  [unwired: 5 in, 6 out]
  }
  n138 = call "Fpga-Uart-State-Machine.vi"("TX FIFO In"=refnum<k21> "HT-UART_TX", "RXD Pin In"=refnum<k21> "UserRTL_microblaze\\uart_rtl_rxd", "RX FIFO In"=refnum<k21> "TH-UART_RX", "TXD Pin In"=refnum<k21> "UserRTL_microblaze\\uart_rtl_txd", "Baud Rate"=w8, "FPGA Clock Rate (MHz)"=u32 100) -> ()  [unwired: 6 in]
  n139 = node-c288(w30) -> ()
  n140 = node-c288() -> (w26:T2)  [unwired: 1 in]
  n141 = timed-loop {
    timing: w26 -> [_]
    timing-out: [_] -> w25
    stop <- _ stop-if-true
    # "Read status signals from the CLIP"
    n142 = xnode "FPGA I/O Node"() -> ("Ethernet\\MgtRefClks_Locked"=→"mgtrefclks_locked":bool, "Ethernet\\MgtRefClks_Valid"=→"mgtrefclks_valid":bool, "Ethernet\\POSC_Complete"=→"posc_complete":bool, "Ethernet\\sPort0_Power_Good"=→"sPort0_Power_Good":bool, "Ethernet\\sPort1_Power_Good"=→"sPort1_Power_Good":bool, "Ethernet\\signal_detect_Port0"=→"signal_detect_Port0":bool, "Ethernet\\signal_detect_Port1"=→"signal_detect_Port1":bool, "Ethernet\\aBlockLockPort0"=→"aBlockLockPort0":bool, "Ethernet\\aBlockLockPort1"=→"aBlockLockPort1":bool)  [unwired: 9 in, 9 out]
  }
  n143 = node-c288(w11) -> ()
  n144 = node-c288(w25) -> ()
  n145 = node-c288(w27) -> ()
  n146 = node-c288(w14) -> ()
  n147 = node-c288(w18) -> ()
  n148 = node-c288(w23) -> ()
